vi "Teleop.vi"(10 "Match Info":T1={"Autonomous Elapsed Seconds"=0.0, "TeleOp Elapsed Seconds"=0.0, "Disabled Elapsed Seconds"=0.0, "Visited Autonomous"=FALSE, "Visited TeleOp"=FALSE, "Visited Disabled"=FALSE, "Autonomous Settings"={"Autonomous Style"=enum."Independent", "VI Refnum"=refnum}}, 11 "Call Context":T2) -> ()   [LabVIEW 2011]
doc: "This VI is called for each TeleOp packet received from the DS where the robot is not disabled. It is often used to read from the joysticks and update I/O or to update setpoints for timed control loops. It should complete and return within 20 milliseconds or it may miss DS packets."
uses:
  <vilib>/Rock Robotics/WPI/DriverStation/WPI_DriverStationDerivedRobotMode.ctl
  <vilib>/Rock Robotics/WPI/DriverStation/WPI_DriverStationMatch Info.ctl
  Robot Global Data.vi
panel:
  out "Position 4":dbl
  out "Position 3":dbl
  out "Shift Control":dbl=2.0 format="%.2f"
  in  "Left High":dbl=0.2
  in  "Right High":dbl=0.8
  in  "Left Mid":dbl=0.25
  in  "Right Mid":dbl=0.7
  in  "Shift Input 2":dbl
  in  "Left Low":dbl=0.8
  in  "Right Low":dbl=0.4
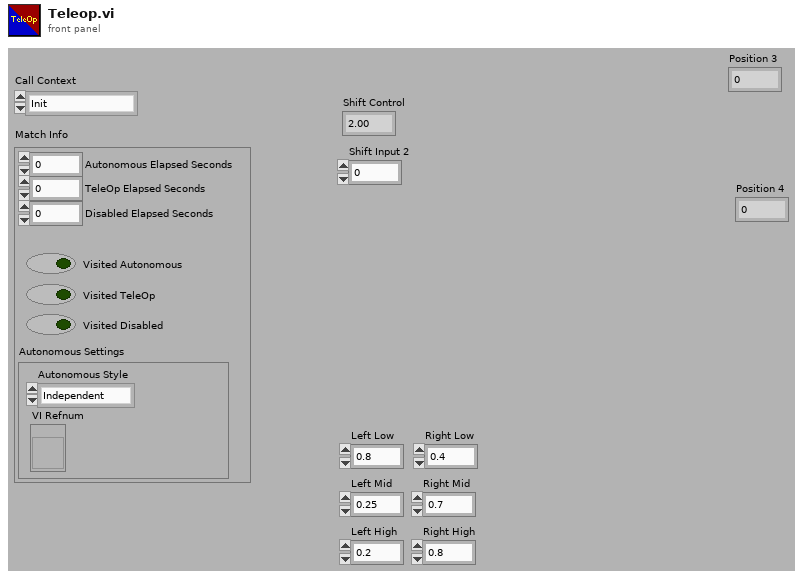
[diagram p1: front panel]
types:
  T1 = typedef "WPI_DriverStationMatch Info.ctl" = cluster{"Autonomous Elapsed Seconds":dbl, "TeleOp Elapsed Seconds":dbl, "Disabled Elapsed Seconds":dbl, "Visited Autonomous":bool, "Visited TeleOp":bool, "Visited Disabled":bool, "Autonomous Settings":cluster{"Autonomous Style":enum16{"Iterative", "Independent"}, "VI Refnum":refnum<vi>}}
  T2 = typedef "WPI_DriverStationDerivedRobotMode.ctl" = enum16{"Init", "Execute", "Stop"}
  T3 = typedef "WPI_JoystickDevRef.ctl" = cluster{"Device":T4}
  T4 = typedef "WPI_JoystickDeviceEnum.ctl" = enum16{"USB 1", "USB 2", "USB 3", "USB 4", "Kinect 1", "Kinect 2"}
  T5 = typedef "WPI_JoystickButtonState.ctl" = cluster{"Button 1":bool, "Button 2":bool, "Button 3":bool, "Button 4":bool, "Button 5":bool, "Button 6":bool, "Button 7":bool, "Button 8":bool, "Button 9":bool, "Button 10":bool, "Button 11":bool, "Button 12":bool}
  T6 = typedef "WPI_MotorControlDeviceRef.ctl" = cluster{"DeviceStatus":errorcluster, "Type":enum16{"PWM", "CAN"}, "PWM":cluster{"Digital Module":T7, "PWM Channel":T8, "DeadBand":T9}, "CAN":cluster{"Device Number":u8, "Control Mode":T10, "Semaphore":T11, "Max Vout":dbl}, "Invert":bool, "TransformRef":T12, "InvTransformRef":T12}
  T7 = typedef "FPGA_TypedefDigitalModule.ctl" = enum16{"Digital Module 1", "Digital Module 2"}
  T8 = typedef "FPGA_DIOPWMChannel.ctl" = enum8{"PWM 1", "PWM 2", "PWM 3", "PWM 4", "PWM 5", "PWM 6", "PWM 7", "PWM 8", "PWM 9", "PWM 10", "Invalid"}
  T9 = typedef "WPI_PWMDeadband.ctl" = cluster{"Name":string, "maxPositivePwm":i32, "minPositivePwm":i32, "centerPwm":i32, "maxNegativePwm":i32, "minNegativePwm":i32, "angularRange":u16}
  T10 = typedef "WPI_CANJaguar_ControlMode.ctl" = enum8{"Percent VBus", "Current", "Speed", "Position", "Voltage"}
  T11 = typedef "Semaphore RefNum" = refnum<k1>
  T12 = typedef "WPI_PWMTransform_ConPane.ctl" = refnum<vi>
  T13 = cluster{"axis 1 (x)":dbl, "axis 2 (y)":dbl, "axis 3 (throttle)":dbl, "axis 4":dbl, "axis 5":dbl, "axis 6":dbl}
  T14 = typedef "WPI_ServoDeviceRef.ctl" = cluster{"DeviceStatus":errorcluster, "Digital Module":T7, "PWM Channel":T8, "DeadBand":T9}
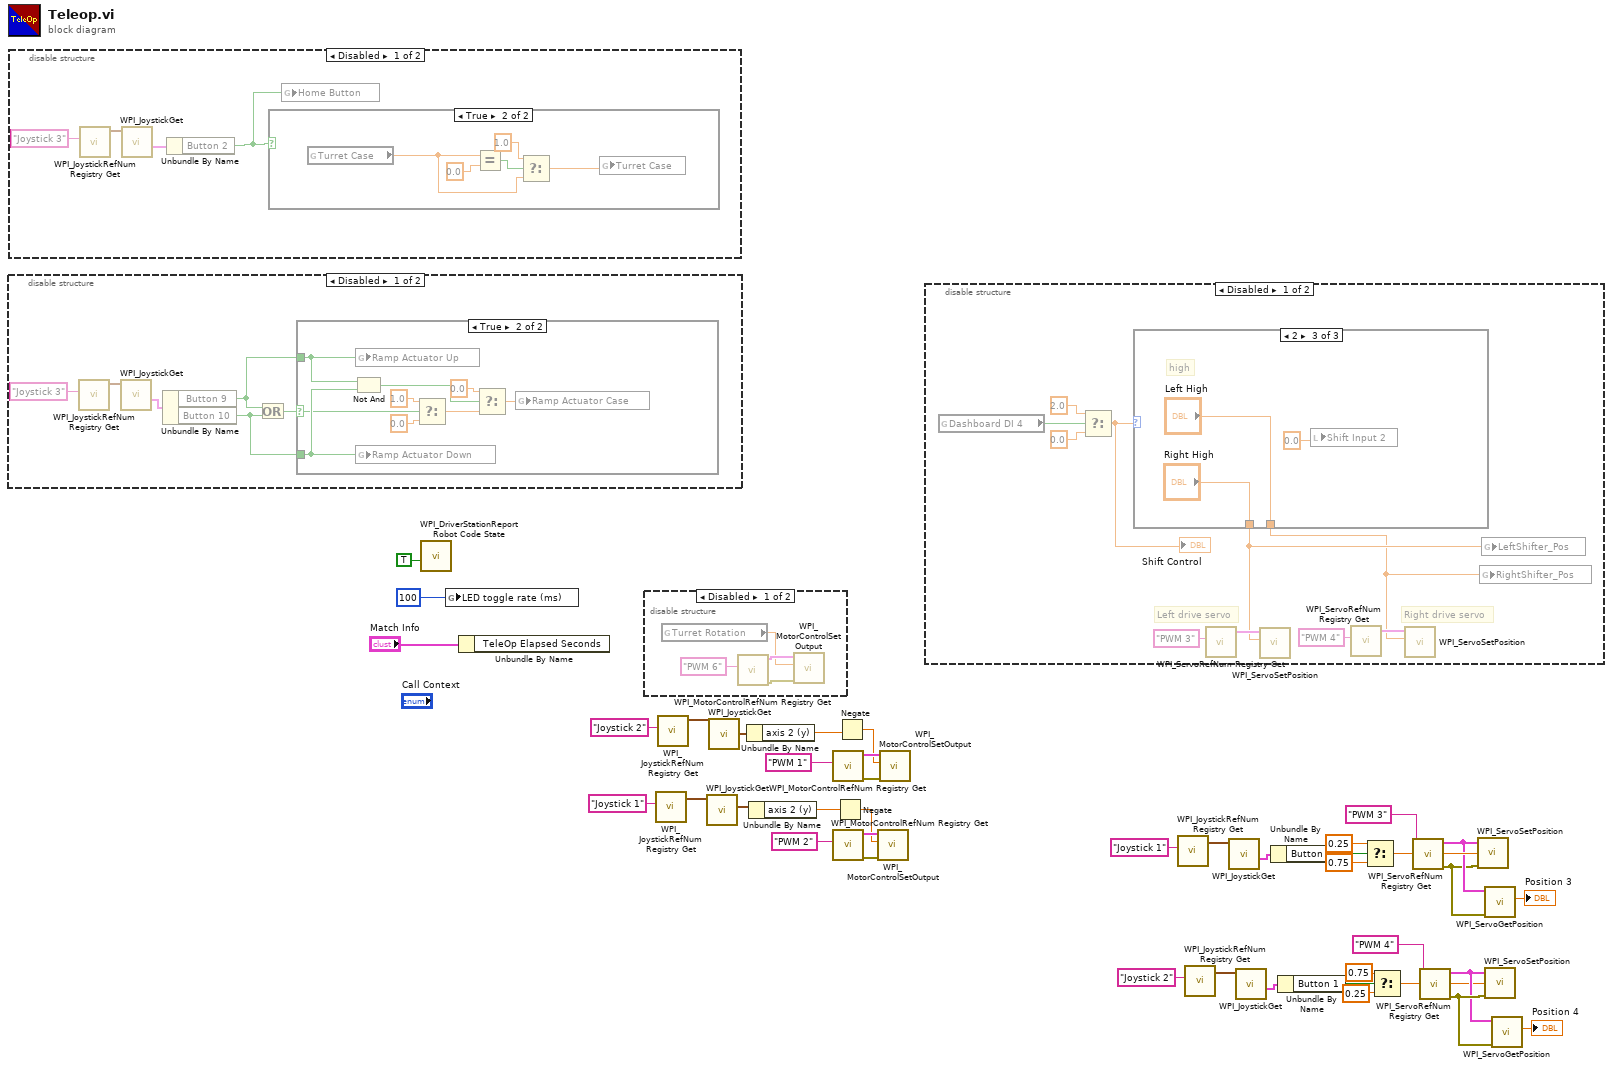
[diagram p0: block diagram]
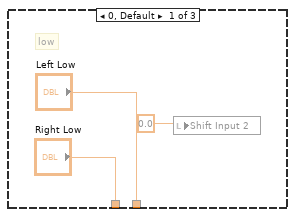
[diagram p7: hidden frame]
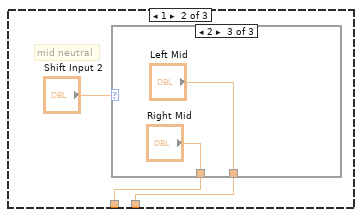
[diagram p8: hidden frame]
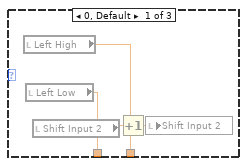
[diagram p9: hidden frame]
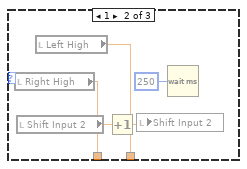
[diagram p10: hidden frame]
diagram:
  n1 = disable-structure shown="Disabled" {
    frame Disabled {
      n2 = call <vilib>:"WPI_JoystickRefNum Registry Get.vi"("refnum name"="Joystick 3") -> ("JoystickDevRef"=w47:T3)  [unwired: 9 in, 1 out]
      n3 = call <vilib>:"WPI_JoystickGet.vi"("JoystickDevRef"=w47) -> ("Buttons"=w46:T5)  [unwired: 4 in, 2 out]
      n4 = Unbundle By Name(w46) -> ("Button 9"=w44:bool, "Button 10"=w43:bool)
      n5 = Or(x=w44, y=w43) -> (x .or. y?=w42:bool)
      n6 = case shown="True" w42 {
        selector: w42 -> [_ w48]
        tunnel: w44 -> [_ w50]
        tunnel: w43 -> [_ w49]
        frame False {
        }
        frame True {
          n7 = Not And(1:w49, 2:w50) -> (0:w51:bool)
          n8 = global write "Robot Global Data.vi" "Ramp Actuator Up"(w50) -> ()
          n9 = global write "Robot Global Data.vi" "Ramp Actuator Down"(w49) -> ()
          n10 = Select(t=1.0, s=w48, f=0.0) -> (s? t:f=w53:dbl)
          n11 = Select(t=0.0, s=w51, f=w53) -> (s? t:f=w56:dbl)
          n12 = global write "Robot Global Data.vi" "Ramp Actuator Case"(w56) -> ()
        }
      }
    }
    frame Enabled {
    }
  }
  n13 = disable-structure shown="Disabled" {
    frame Disabled {
      n14 = call <vilib>:"WPI_JoystickRefNum Registry Get.vi"("refnum name"="Joystick 3") -> ("JoystickDevRef"=w58:T3)  [unwired: 9 in, 1 out]
      n15 = call <vilib>:"WPI_JoystickGet.vi"("JoystickDevRef"=w58) -> ("Buttons"=w59:T5)  [unwired: 4 in, 2 out]
      n16 = Unbundle By Name(w59) -> ("Button 2"=w57:bool)
      n17 = case shown="True" w57 {
        frame False {
        }
        frame True {
          n18 = global read "Robot Global Data.vi" "Turret Case"() -> (w62:dbl)
          n19 = Equal?(x=w62, y=0.0) -> (x = y?=w64:bool)
          n20 = Select(t=1.0, s=w64, f=w62) -> (s? t:f=w61:dbl)
          n21 = global write "Robot Global Data.vi" "Turret Case"(w61) -> ()
        }
      }
      n22 = global write "Robot Global Data.vi" "Home Button"(w57) -> ()
    }
    frame Enabled {
    }
  }
  n23 = call <vilib>:"WPI_DriverStationReport Robot Code State.vi"("TeleOp"=TRUE ("Autonomous")) -> ()  [unwired: 10 in, 1 out]
  n24 = global write "Robot Global Data.vi" "LED toggle rate (ms)"(u32 100 ("LED ms toggle rate")) -> ()
  n25 = Unbundle By Name("Match Info") -> ()  [unwired: 1 out]
  n26 = disable-structure shown="Disabled" {
    frame Disabled {
      n27 = global read "Robot Global Data.vi" "Turret Rotation"() -> (w66:dbl)
      n28 = call <vilib>:"WPI_MotorControlRefNum Registry Get.vi"("refnum name"="PWM 6") -> ("error out"=w69:errorcluster, "MotorControlDevRef"=w68:T6)  [unwired: 9 in]
      n29 = call <vilib>:"WPI_MotorControlSetOutput.vi"("error in (no error)"=w69, "Output"=w66, "MotorControlDevRef"=w68) -> ()  [unwired: 7 in, 2 out]
    }
    frame Enabled {
    }
  }
  n30 = call <vilib>:"WPI_JoystickRefNum Registry Get.vi"("refnum name"="Joystick 1") -> ("JoystickDevRef"=w33:T3)  [unwired: 9 in, 1 out]
  n31 = call <vilib>:"WPI_JoystickRefNum Registry Get.vi"("refnum name"="Joystick 2") -> ("JoystickDevRef"=w36:T3)  [unwired: 9 in, 1 out]
  n32 = call <vilib>:"WPI_JoystickGet.vi"("JoystickDevRef"=w33) -> ("Axes"=w37:T13)  [unwired: 4 in, 2 out]
  n33 = call <vilib>:"WPI_JoystickGet.vi"("JoystickDevRef"=w36) -> ("Axes"=w38:T13)  [unwired: 4 in, 2 out]
  n34 = Unbundle By Name(w38) -> ("axis 2 (y)"=w26:dbl)
  n35 = Unbundle By Name(w37) -> ("axis 2 (y)"=w24:dbl)
  n36 = call <vilib>:"WPI_MotorControlRefNum Registry Get.vi"("refnum name"="PWM 1") -> ("error out"=w30:errorcluster, "MotorControlDevRef"=w29:T6)  [unwired: 9 in]
  n37 = call <vilib>:"WPI_MotorControlRefNum Registry Get.vi"("refnum name"="PWM 2") -> ("error out"=w32:errorcluster, "MotorControlDevRef"=w31:T6)  [unwired: 9 in]
  n38 = Negate(x=w24) -> (-x=w23:dbl)
  n39 = Negate(x=w26) -> (-x=w25:dbl)
  n40 = call <vilib>:"WPI_MotorControlSetOutput.vi"("error in (no error)"=w32, "Output"=w23, "MotorControlDevRef"=w31) -> ()  [unwired: 7 in, 2 out]
  n41 = call <vilib>:"WPI_MotorControlSetOutput.vi"("error in (no error)"=w30, "Output"=w25, "MotorControlDevRef"=w29) -> ()  [unwired: 7 in, 2 out]
  n42 = disable-structure shown="Disabled" {
    frame Disabled {
      # "Right drive servo"
      # "Left drive servo"
      n43 = global read "Robot Global Data.vi" "Dashboard DI 4"() -> (w72:bool)
      n44 = Select(t=2.0, s=w72, f=0.0) -> (s? t:f=w74:dbl)
      "Shift Control" <- w74
      n45 = case shown="2" w74 {
        tunnel: ["Left Low" w84 "Left High"] -> w70
        tunnel: ["Right Low" w83 "Right High"] -> w71
        frame 0, Default {
          # "low"
          n46 = local write "Shift Input 2"(0.0 ("Input 2")) -> ()
        }
        frame 1 {
          # "mid neutral"
          n47 = case shown="2" "Shift Input 2" {
            tunnel: [w89 w90 "Left Mid"] -> w84
            tunnel: [w88 w91 "Right Mid"] -> w83
            frame 0, Default {
              n48 = local read "Left High"() -> (w89:dbl)
              n49 = local read "Left Low"() -> (w88:dbl)
              n50 = local read "Shift Input 2"() -> (w87:dbl)
              n51 = Increment(x=w87) -> (x+1=w86:dbl)
              n52 = local write "Shift Input 2"(w86) -> ()
            }
            frame 1 {
              n53 = local read "Right High"() -> (w91:dbl)
              n54 = local read "Shift Input 2"() -> (w93:dbl)
              n55 = local read "Left High"() -> (w90:dbl)
              n56 = Increment(x=w93) -> (x+1=w92:dbl)
              n57 = local write "Shift Input 2"(w92) -> ()
              n58 = Wait (ms)(milliseconds to wait=u32 250) -> ()  [unwired: 1 out]
            }
            frame 2 {
            }
          }
        }
        frame 2 {
          # "high"
          n59 = local write "Shift Input 2"(0.0 ("Input 2")) -> ()
        }
      }
      n60 = call <vilib>:"WPI_ServoRefNum Registry Get.vi"("refnum name"="PWM 3") -> ("ServoDeviceRef"=w79:T14)  [unwired: 1 in, 9 out]
      n61 = call <vilib>:"WPI_ServoSetPosition.vi"("Position"=w71, "ServoDeviceRef"=w79) -> ()  [unwired: 1 in, 9 out]
      n62 = call <vilib>:"WPI_ServoRefNum Registry Get.vi"("refnum name"="PWM 4") -> ("ServoDeviceRef"=w75:T14)  [unwired: 1 in, 9 out]
      n63 = call <vilib>:"WPI_ServoSetPosition.vi"("Position"=w70, "ServoDeviceRef"=w75) -> ()  [unwired: 1 in, 9 out]
      n64 = global write "Robot Global Data.vi" "RightShifter_Pos"(w70) -> ()
      n65 = global write "Robot Global Data.vi" "LeftShifter_Pos"(w71) -> ()
    }
    frame Enabled {
    }
  }
  n66 = call <vilib>:"WPI_JoystickRefNum Registry Get.vi"("refnum name"="Joystick 1") -> ("JoystickDevRef"=w22:T3)  [unwired: 9 in, 1 out]
  n67 = call <vilib>:"WPI_JoystickRefNum Registry Get.vi"("refnum name"="Joystick 2") -> ("JoystickDevRef"=w1:T3)  [unwired: 9 in, 1 out]
  n68 = call <vilib>:"WPI_JoystickGet.vi"("JoystickDevRef"=w22) -> ("Buttons"=w20:T5)  [unwired: 4 in, 2 out]
  n69 = call <vilib>:"WPI_JoystickGet.vi"("JoystickDevRef"=w1) -> ("Buttons"=w3:T5)  [unwired: 4 in, 2 out]
  n70 = Unbundle By Name(w20) -> ("Button 1"=w19:bool)
  n71 = Unbundle By Name(w3) -> ("Button 1"=w4:bool)
  n72 = Select(t=0.25, s=w19, f=0.75) -> (s? t:f=w16:dbl)
  n73 = Select(t=0.75, s=w4, f=0.25) -> (s? t:f=w7:dbl)
  n74 = call <vilib>:"WPI_ServoRefNum Registry Get.vi"("refnum name"="PWM 3") -> ("error out"=w13:errorcluster, "ServoDeviceRef"=w14:T14)  [unwired: 9 in]
  n75 = call <vilib>:"WPI_ServoRefNum Registry Get.vi"("refnum name"="PWM 4") -> ("error out"=w10:errorcluster, "ServoDeviceRef"=w9:T14)  [unwired: 9 in]
  n76 = call <vilib>:"WPI_ServoSetPosition.vi"("error in (no error)"=w13, "Position"=w16, "ServoDeviceRef"=w14) -> ()  [unwired: 7 in, 2 out]
  n77 = call <vilib>:"WPI_ServoGetPosition.vi"("error in (no error)"=w13, "ServoDeviceRef"=w14) -> ("Position"=→"Position 3":dbl)  [unwired: 7 in, 2 out]
  n78 = call <vilib>:"WPI_ServoSetPosition.vi"("error in (no error)"=w10, "Position"=w7, "ServoDeviceRef"=w9) -> ()  [unwired: 7 in, 2 out]
  n79 = call <vilib>:"WPI_ServoGetPosition.vi"("error in (no error)"=w10, "ServoDeviceRef"=w9) -> ("Position"=→"Position 4":dbl)  [unwired: 7 in, 2 out]
